vi "ID Query.vi"(8 "error in (no error)":errorcluster, 9 "timeout ms (55000)":i32=55000, 11 "VISA resource name":refnum<visa-resource-name>) -> (0 "error out":errorcluster, 1 "Serial":i32, 2 "Model Name":string, 3 "VISA resource name out":refnum<visa-resource-name>)   [LabVIEW 2011, in "Ocean Server OS4000.lvlib"]
doc: "Queries for the identification information of the instrument."
uses:
  Ocean Server OS4000.lvlib
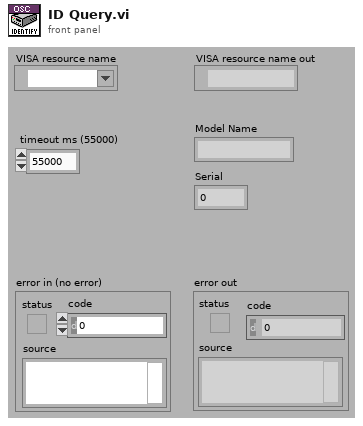
[diagram p1: front panel]
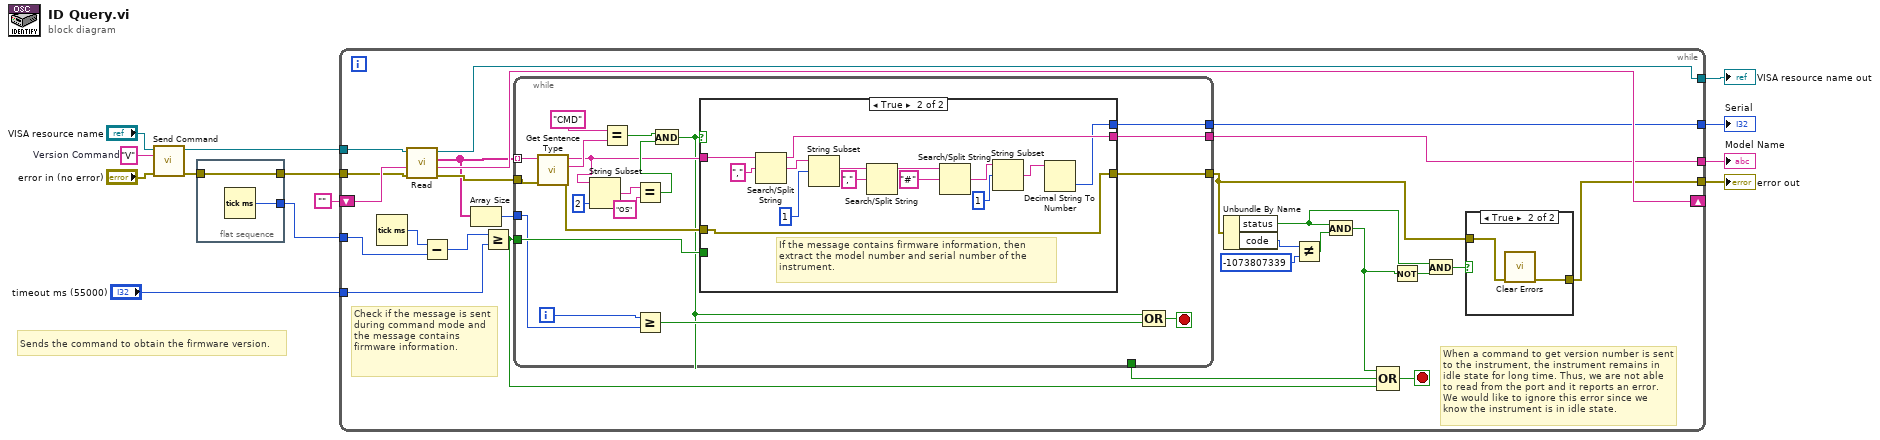
[diagram p0: block diagram]
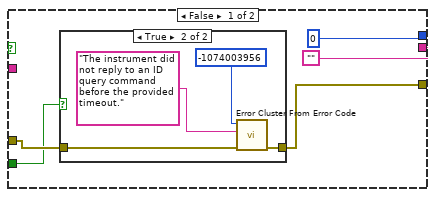
[diagram p2: hidden frame]
diagram:
  w9 = "V"  # Version Command
  # "Sends the command to obtain the firmware version."
  n1 = call "Send Command.vi"("error in (no error)"="error in (no error)", "Message"=w9, "VISA resource name"="VISA resource name") -> ("error out"=w3:errorcluster, "VISA resource out"=w7:refnum<visa-resource-name>)  [unwired: 7 in]
  n2 = flat-sequence {
    tunnel: w3 -> [w15]
    tunnel: [w15] -> w5
    tunnel: [w14] -> w12
    frame #0 {
      n3 = Tick Count (ms)() -> (millisecond timer value=w14:u32)
    }
  }
  n4 = while {
    tunnel: w7 -> [w36]
    tunnel: [w35] -> w13
    shift-right: [w33] -> _
    shift-left: "" ("Remaining Sentence") -> [w34]
    tunnel: w12 -> [w40]
    tunnel: "timeout ms (55000)" -> [w38]
    tunnel: w5 -> [w26]
    tunnel: [w20] -> w4
    tunnel: [w17] -> w2
    tunnel: [w16] -> w1
    stop <- w37 stop-if-true
    # "When a command to get version number is sent to the instrument, the instrument remains in idle state for long time. Thus, we are not able to read from the port and it reports an error. We would like to ignore this error since we know the instrument is in idle state."
    # "Check if the message is sent during command mode and the message contains firmware information."
    n5 = Tick Count (ms)() -> (millisecond timer value=w41:u32)
    n6 = call "Read.vi"("error in (no error)"=w26, "Text to prepend to sentence"=w34, "VISA resource name"=w36) -> ("error out"=w32:errorcluster, "Remaining Sentence"=w33:string, "Ocean Server Sentences"=w19:string[], "VISA resource name out"=w35:refnum<visa-resource-name>)  [unwired: 5 in]
    n7 = Subtract(x=w41, y=w40) -> (x-y=w39:u32)
    n8 = Array Size(array=w19) -> (size(s)=w18:i32)
    n9 = Greater Or Equal?(x=w39, y=w38) -> (x >= y?=w27:bool)
    n10 = while {
      tunnel: w19 -> [w61] mode=indexing
      tunnel: w32 -> [w59]
      tunnel: [w45] -> w31
      tunnel: w27 -> [w51]
      tunnel: [w50] -> w21
      tunnel: w18 -> [w48]
      tunnel: [w43] -> w17
      tunnel: [w42] -> w16
      i -> [w47]
      stop <- w44 stop-if-true
      n11 = call "Get Sentence Type.vi"("error in (no error)"=w59, "Sentence In"=w61) -> ("error out"=w49:errorcluster, "Sentence Type"=w58:string, "Sentence Out"=w52:string)  [unwired: 7 in]
      n12 = String Subset(string=w52, length (rest)=2 ("length (rest)")) -> (substring=w56:string)  [unwired: 1 in]
      n13 = Equal?(x="CMD", y=w58) -> (x = y?=w53:bool)
      n14 = Equal?(x=w56, y="OS") -> (x = y?=w54:bool)
      n15 = Greater Or Equal?(x=w47, y=w48) -> (x >= y?=w46:bool)
      n16 = And(x=w53, y=w54) -> (x .and. y?=w45:bool)
      n17 = case shown="True" w45 {
        tunnel: w52 -> [_ w85]
        tunnel: w49 -> [w66 w78]
        tunnel: [w65 w78] -> w50
        tunnel: w51 -> [w64 _]
        tunnel: ["" w73] -> w43
        tunnel: [0 w72] -> w42
        frame False {
          n18 = case shown="True" w64 {
            tunnel: [w67 w71] -> w65
            tunnel: w66 -> [w67 w70]
            frame False {
            }
            frame True {
              n19 = call <vilib>:"Error Cluster From Error Code.vi"("error in (no error)"=w70, "error message (\"\")"="The instrument did not reply to an ID query command before the provided timeout." ("[error source] (\" \")"), "error code (0)"=-1074003956 ("[error code] (0)")) -> ("error out"=w71:errorcluster)  [unwired: 6 in]
            }
          }
        }
        frame True {
          # "If the message contains firmware information, then extract the model number and serial number of the instrument."
          n20 = Search/Split String(string=w85, search string/char (-)=",") -> (substring before match=w73:string, match + rest of string=w76:string)  [unwired: 1 in, 1 out]
          n21 = String Subset(string=w76, offset (0)=1) -> (substring=w75:string)  [unwired: 1 in]
          n22 = Search/Split String(string=w75, search string/char (-)=",") -> (substring before match=w82:string)  [unwired: 1 in, 2 out]
          n23 = Search/Split String(string=w82, search string/char (-)="#") -> (match + rest of string=w80:string)  [unwired: 1 in, 2 out]
          n24 = String Subset(string=w80, offset (0)=1) -> (substring=w77:string)  [unwired: 1 in]
          n25 = Decimal String To Number(string=w77) -> (number=w72:i32)  [unwired: 2 in, 1 out]
        }
      }
      n26 = Compound Arithmetic op=OR(w45, w46) -> (w44:bool)
    }
    n27 = Unbundle By Name(w21) -> ("status"=w24:bool, "code"=w30:i32)
    n28 = Not Equal?(x=w30, y=-1073807339) -> (x != y?=w28:bool)
    n29 = And(x=w24, y=w28) -> (x .and. y?=w22:bool)
    n30 = Compound Arithmetic op=OR(w22, w31, w27) -> (w37:bool)
    n31 = Not(x=w22) -> (.not. x?=w23:bool)
    n32 = And(x=w24, y=w23) -> (x .and. y?=w25:bool)
    n33 = case shown="True" w25 {
      tunnel: w21 -> [w86 w88]
      tunnel: [w86 w87] -> w20
      frame False {
      }
      frame True {
        n34 = call <vilib>:"Clear Errors.vi"("error in (no error)"=w88) -> ("error out"=w87:errorcluster)  [unwired: 6 in]
      }
    }
  }
  "VISA resource name out" <- w13
  "error out" <- w4
  "Model Name" <- w2
  "Serial" <- w1
